vi "Charging_Set MICS Globals.vi"(4 "error in":errorcluster, 7 "MICS inputs":T1={"address"="COM14", "chan"=1, "ID"=4417} {"ID" format="%04x"; "chan" min=1 max=10 step=1}) -> (0 "error out":errorcluster, 3 "address":refnum<visa-resource-name>="COM14")   [LabVIEW 2020]
uses:
  Telemetry/MICS_ID Global.vi
  Telemetry/MICS_Channel Global.vi
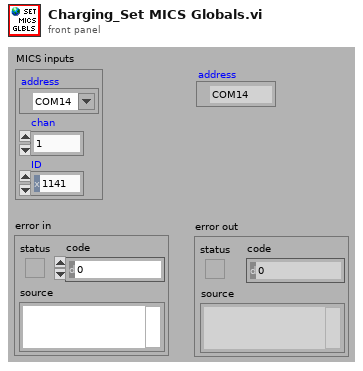
[diagram p1: front panel]
types:
  T1 = cluster{"address":refnum<visa-resource-name>, "chan":u16, "ID":u32}
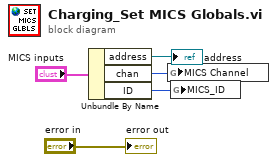
[diagram p0: block diagram]
diagram:
  n1 = Unbundle By Name("MICS inputs") -> ("address"=→"address":refnum<visa-resource-name>, "chan"=w3:u16, "ID"=w2:u32)
  n2 = global write "MICS_Channel Global.vi" "MICS Channel"(w3) -> ()
  n3 = global write "MICS_ID Global.vi" "MICS_ID"(w2) -> ()
  "error out" <- "error in"
